vi "String Limit Example.vi"() -> ()   [LabVIEW 2009]
uses:
  String_XControl.xctl
panel:
  in  "String Length":i32=10
  in  "Stop":bool
  in  "String_XControl":string(xcontrol)
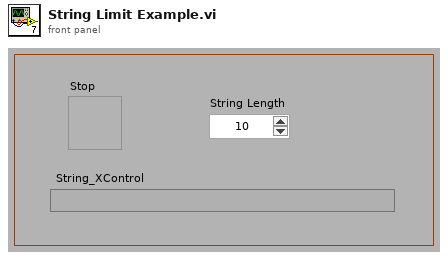
[diagram p1: front panel]
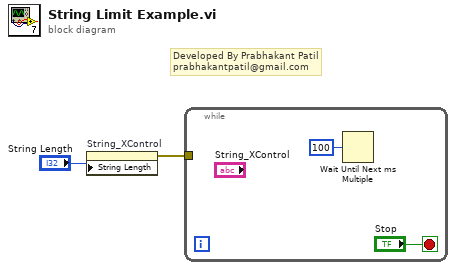
[diagram p0: block diagram]
diagram:
  # "Developed By Prabhakant Patil\nprabhakantpatil@gmail.com"
  n1 = property on="String_XControl" class="String_XControl (strict)"("String Length"="String Length") -> (error out=w2:errorcluster)  [unwired: 2 in, 1 out]
  n2 = while {
    tunnel: w2 -> [_]
    stop <- "Stop" stop-if-true
    n3 = Wait Until Next ms Multiple(millisecond multiple=u32 100) -> ()  [unwired: 1 out]
  }
